vi "tabRecurser.vi"(4 "examineArrays?(T)":bool, 6 "Mode":enum16{"Read", "Write"}(ring)=enum."Write", 7 "controlsOnly":bool, 9 "SectionNameIn":string, 10 "controlsIn[]":refnum<vi>[](array[refnum]), 11 "INIrefnumIn":T3) -> (1 "varDescriptions":T1[](array[typedef]), 3 "INIrefnumOut":T3)   [LabVIEW 2021]
uses:
  <vilib>/Utility/config.llb/Config Data RefNum.ctl
  varDescriptor.ctl
  <vilib>/Utility/Data Type/Type Definitions/Data Type.ctl
  <vilib>/Utility/Data Type/NI_Data Type.lvlib
  <vilib>/Utility/config.llb/NI_LVConfig.lvlib
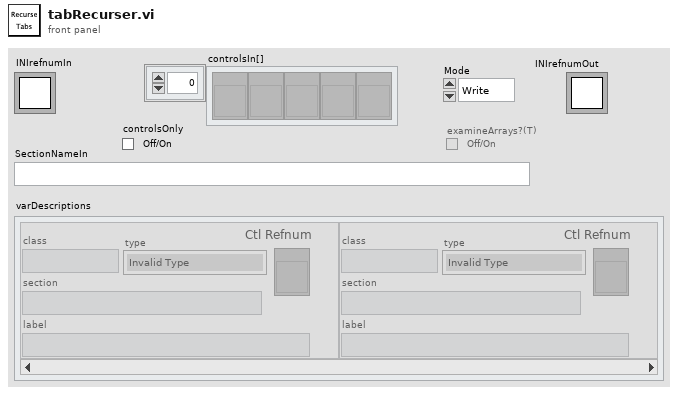
[diagram p1: front panel]
types:
  T1 = typedef "varDescriptor.ctl" = cluster{"class":string, "type":T2, "section":string, "label":string, "Ctl Refnum":refnum<vi>}
  T2 = typedef "NI_Data Type.lvlib/Data Type.ctl" = enum8{"Invalid Type", "Void", "I8", "I16", "I32", "I64", "U8", "U16", "U32", "U64", "Single Float", "Double Float", "Extended Float", "Single Complex", "Double Complex", "Extended Complex", "Enum U8", "Enum U16", "Enum U32", "Enum U64", "Single Float With Unit", "Double Float With Unit", "Extended Float With Unit", "Single Complex with Unit", "Double Complex with Unit", "Extended Complex with Unit", "Boolean", "String", "Path", "Picture", "Tag", "Array", "Cluster", "Variant", "LV Variant", "Waveform", "Timestamp", "Digital Waveform", "Digital Data", "ExpressData", "Refnum", "External Data", "VI", "Poly VI", "LabVIEW Class Instance", "Fixed Point", "Set Collection", "Map Collection"}
  T3 = typedef "NI_LVConfig.lvlib/Config Data RefNum.ctl" = refnum<k1>
  T4 = cluster{"ClassName":string, "type":T2, "SectionNameIn":string, "name":string, refnum<vi>}
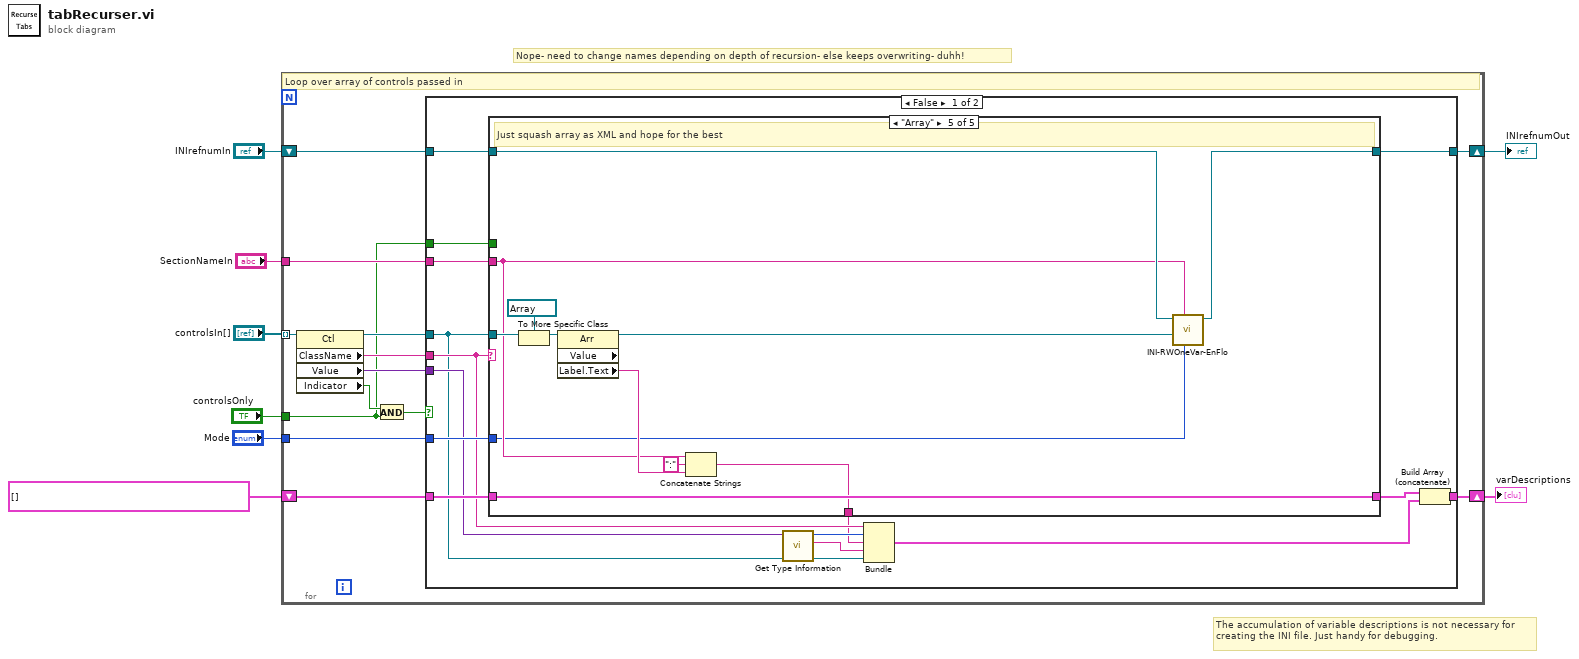
[diagram p0: block diagram]
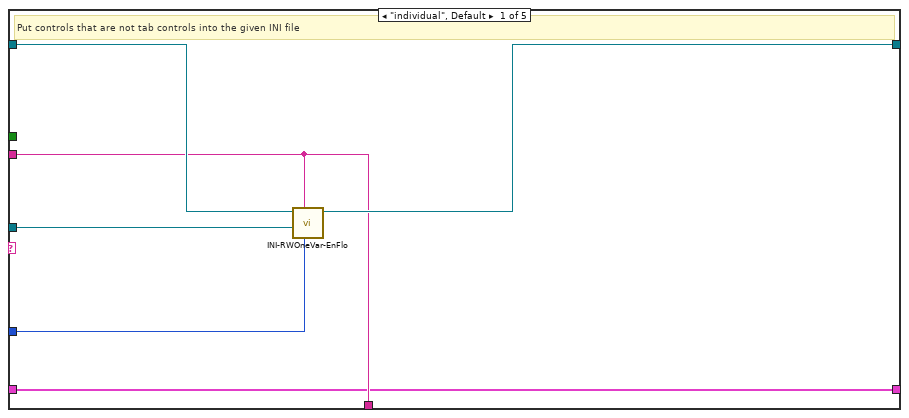
[diagram p2: hidden frame]
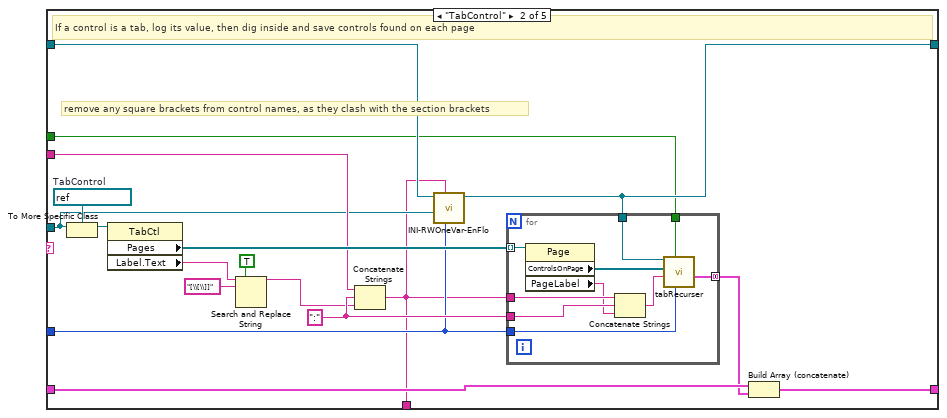
[diagram p3: hidden frame]
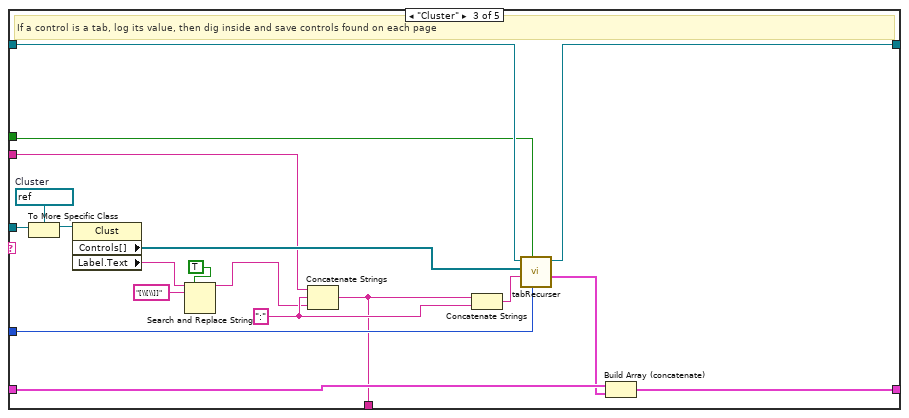
[diagram p4: hidden frame]
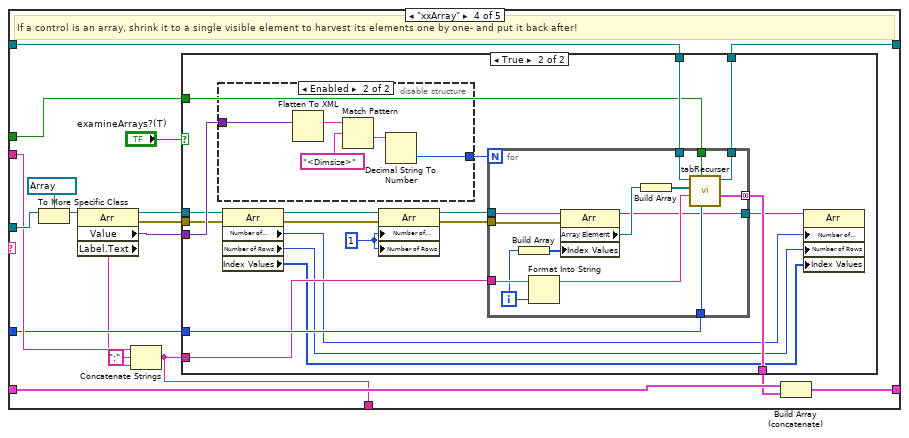
[diagram p5: hidden frame]
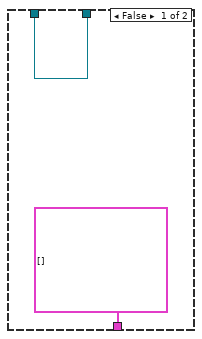
[diagram p6: hidden frame]
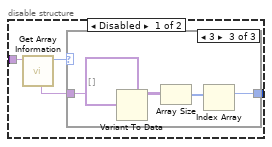
[diagram p7: hidden frame]
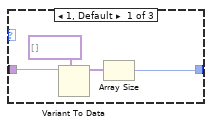
[diagram p8: hidden frame]
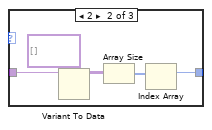
[diagram p9: hidden frame]
diagram:
  # "Nope- need to change names depending on depth of recursion- else keeps overwriting- duhh!"
  # "The accumulation of variable descriptions is not necessary for creating the INI file. Just handy for debugging."
  n1 = for {
    tunnel: "controlsIn[]" -> [w21] mode=indexing
    shift-right: [w13] -> w3
    shift-left: T1[] [] ("Array 2") -> [w20]
    tunnel: "SectionNameIn" -> [w19]
    shift-right: [w17] -> w5
    shift-left: "INIrefnumIn" -> [w18]
    tunnel: "Mode" -> [w16]
    tunnel: "controlsOnly" -> [w9]
    # "Loop over array of controls passed in"
    n2 = property class="Ctl"(reference=w21) -> (reference out=w12:refnum<vi>, "ClassName"=w14:string, "Value"=w15:variant, "Indicator"=w11:bool)  [unwired: 1 in, 1 out]
    n3 = And(x=w11, y=w9) -> (x .and. y?=w10:bool)
    n4 = case shown="False" w10 {
      tunnel: w20 -> [w35 w177]
      tunnel: w19 -> [w34 _]
      tunnel: w18 -> [w33 w178]
      tunnel: [w32 w178] -> w17
      tunnel: w16 -> [w31 _]
      tunnel: w15 -> [w28 _]
      tunnel: w14 -> [w27 _]
      tunnel: [w26 w177] -> w13
      tunnel: w12 -> [w24 _]
      tunnel: w9 -> [w22 _]
      frame False {
        n5 = case shown="\"Array\"" w27 {
          tunnel: w24 -> [w42 w52 w80 w106 w175]
          tunnel: [w37 w59 w88 w104 w174] -> w36
          tunnel: w35 -> [w37 w60 w89 w105 w174]
          tunnel: w34 -> [w38 w55 w83 w102 w167]
          tunnel: w33 -> [w41 w53 w81 w100 w172]
          tunnel: [w40 w48 w84 w98 w171] -> w32
          tunnel: w31 -> [w39 w51 w79 w101 w165]
          tunnel: [w38 w49 w77 w97 w170] -> w23
          tunnel: w22 -> [_ w43 w71 w90 _]
          frame "individual", Default {
            # "Put controls that are not tab controls into the given INI file"
            n6 = call "INI-RWOneVar-EnFlo.vi"("Mode"=w39, "section"=w38, "controlRefIn"=w42, "INIfileRefIn"=w41) -> ("INIfileRefOut"=w40:T3)  [unwired: 6 in, 1 out]
          }
          frame "TabControl" {
            w54 = ":" ("string")
            w56 = refnum<vi> refnum  # TabControl
            # "remove any square brackets from control names, as they clash with the section brackets"
            # "If a control is a tab, log its value, then dig inside and save controls found on each page"
            n7 = To More Specific Class(target class=w56, reference=w52) -> (specific class reference=w58:refnum<vi>)  [unwired: 1 in, 1 out]
            n8 = property class="TabCtl"(reference=w58) -> ("Pages"=w57:refnum<vi>[], "Label.Text"=w46:string)  [unwired: 1 in, 2 out]
            n9 = Search and Replace String(replace all?=TRUE ("replace all? (F)"), input string=w46, search string="[\\[\\]]") -> (result string=w45:string)  [unwired: 5 in, 3 out]
            n10 = Concatenate Strings(w55, w54, w45) -> (w49:string)
            n11 = call "INI-RWOneVar-EnFlo.vi"("Mode"=w51, "section"=w49, "controlRefIn"=w52, "INIfileRefIn"=w53) -> ("INIfileRefOut"=w48:T3)  [unwired: 6 in, 1 out]
            n12 = for {
              tunnel: w57 -> [w70] mode=indexing
              tunnel: w49 -> [w66]
              tunnel: w48 -> [w68]
              tunnel: w51 -> [w67]
              tunnel: w54 -> [w65]
              tunnel: [w62] -> w50 mode=concatenating
              tunnel: w43 -> [w61]
              n13 = property class="Page"(reference=w70) -> ("ControlsOnPage"=w69:refnum<vi>[], "PageLabel"=w64:string)  [unwired: 1 in, 2 out]
              n14 = Concatenate Strings(w66, w65, w64) -> (w63:string)
              n15 = call "tabRecurser.vi"("Mode"=w67, "controlsOnly"=w61, "SectionNameIn"=w63, "controlsIn[]"=w69, "INIrefnumIn"=w68) -> ("varDescriptions"=w62:T1[])  [unwired: 5 in, 1 out]
            }
            n16 = Build Array (concatenate)(w60, w50) -> (w59:T1[])
          }
          frame "Cluster" {
            w82 = ":" ("string")
            w85 = refnum<vi> refnum  # Cluster
            # "If a control is a tab, log its value, then dig inside and save controls found on each page"
            n17 = To More Specific Class(target class=w85, reference=w80) -> (specific class reference=w87:refnum<vi>)  [unwired: 1 in, 1 out]
            n18 = property class="Clust"(reference=w87) -> ("Controls[]"=w86:refnum<vi>[], "Label.Text"=w73:string)  [unwired: 1 in, 2 out]
            n19 = Search and Replace String(replace all?=TRUE ("replace all? (F)"), input string=w73, search string="[\\[\\]]") -> (result string=w72:string)  [unwired: 5 in, 3 out]
            n20 = Concatenate Strings(w83, w82, w72) -> (w77:string)
            n21 = Concatenate Strings(w77, w82) -> (w76:string)
            n22 = call "tabRecurser.vi"("Mode"=w79, "controlsOnly"=w71, "SectionNameIn"=w76, "controlsIn[]"=w86, "INIrefnumIn"=w81) -> ("varDescriptions"=w78:T1[], "INIrefnumOut"=w84:T3)  [unwired: 5 in]
            n23 = Build Array (concatenate)(w89, w78) -> (w88:T1[])
          }
          frame "xxArray" {
            # "If a control is an array, shrink it to a single visible element to harvest its elements one by one- and put it back after!"
            n24 = To More Specific Class(target class=refnum<vi> refnum ("Cluster-Array"), reference=w106) -> (specific class reference=w96:refnum<vi>)  [unwired: 1 in, 1 out]
            n25 = property class="Arr"(reference=w96) -> (reference out=w93:refnum<vi>, error out=w92:errorcluster, "Value"=w94:variant, "Label.Text"=w95:string)  [unwired: 1 in]
            n26 = Concatenate Strings(w102, ":" ("string"), w95) -> (w97:string)
            n27 = case shown="True" "examineArrays?(T)" {
              tunnel: w101 -> [_ w128]
              tunnel: w100 -> [w109 w127]
              tunnel: [T1[] [] ("varDescriptions") w126] -> w99
              tunnel: [w109 w125] -> w98
              tunnel: w97 -> [_ w124]
              tunnel: w94 -> [_ w122]
              tunnel: w93 -> [_ w121]
              tunnel: w92 -> [_ w118]
              tunnel: w90 -> [_ w110]
              frame False {
              }
              frame True {
                w115 = u32 1 ("Number of Columns")
                n28 = disable-structure shown="Enabled" {
                  disable-tunnel: [w131 w146] -> w123
                  disable-tunnel: w122 -> [w130 w147]
                  frame Disabled {
                    n29 = call <vilib>:"Get Array Information.vi"("variant"=w130) -> ("number of dimensions"=w129:i32)  [unwired: 7 in, 3 out]
                    n30 = case shown="3" w129 {
                      tunnel: w130 -> [w134 w139 w144]
                      tunnel: [w132 w136 w141] -> w131
                      frame 1, Default {
                        n31 = Variant To Data(type=variant[] [], Variant=w134) -> (data=w133:variant[])  [unwired: 1 in, 1 out]
                        n32 = Array Size(array=w133) -> (size(s)=w132:i32)
                      }
                      frame 2 {
                        n33 = Variant To Data(type=variant[][] [], Variant=w139) -> (data=w138:variant[][])  [unwired: 1 in, 1 out]
                        n34 = Array Size(array=w138) -> (size(s)=w137:i32[])
                        n35 = Index Array(array=w137) -> (element=w136:i32)  [unwired: 1 in]
                      }
                      frame 3 {
                        n36 = Variant To Data(type=variant[][][] [], Variant=w144) -> (data=w143:variant[][][])  [unwired: 1 in, 1 out]
                        n37 = Array Size(array=w143) -> (size(s)=w142:i32[])
                        n38 = Index Array(array=w142) -> (element=w141:i32)  [unwired: 1 in]
                      }
                    }
                  }
                  frame Enabled {
                    n39 = Flatten To XML(6:w147) -> (2:w148:string)
                    n40 = Match Pattern(string=w148, regular expression="<Dimsize>") -> (after substring=w150:string)  [unwired: 1 in, 3 out]
                    n41 = Decimal String To Number(string=w150) -> (number=w146:i32)  [unwired: 2 in, 1 out]
                  }
                }
                n42 = property class="Arr"(reference=w121, error in=w118) -> (reference out=w120:refnum<vi>, error out=w119:errorcluster, "Number of Columns"=w113:u32, "Number of Rows"=w112:u32, "Index Values"=w111:u32[])
                n43 = property class="Arr"(reference=w120, error in=w119, "Number of Columns"=w115, "Number of Rows"=w115) -> (reference out=w117:refnum<vi>, error out=w116:errorcluster)
                n44 = for {
                  N: w123 -> [_]
                  tunnel: w116 -> [w156]
                  tunnel: w117 -> [w157]
                  tunnel: w128 -> [w164]
                  tunnel: w127 -> [w163]
                  tunnel: [w162] -> w126 mode=concatenating
                  tunnel: [w161] -> w125
                  tunnel: w124 -> [w160]
                  tunnel: [w152] -> w114
                  tunnel: w110 -> [w151]
                  i -> [w155]
                  n45 = Build Array(w155) -> (w154:i32[])
                  n46 = Format Into String(initial string=w160, w155) -> (resulting string=w159:string)  [unwired: 2 in, 1 out]
                  n47 = property class="Arr"(reference=w157, error in=w156, "Index Values"=w154) -> (reference out=w152:refnum<vi>, "Array Element"=w153:refnum<vi>)  [unwired: 1 out]
                  n48 = Build Array(w153) -> (w158:refnum<vi>[])
                  n49 = call "tabRecurser.vi"("Mode"=w164, "controlsOnly"=w151, "SectionNameIn"=w159, "controlsIn[]"=w158, "INIrefnumIn"=w163) -> ("varDescriptions"=w162:T1[], "INIrefnumOut"=w161:T3)  [unwired: 5 in]
                }
                n50 = property class="Arr"(reference=w114, "Number of Columns"=w113, "Number of Rows"=w112, "Index Values"=w111) -> ()  [unwired: 1 in, 2 out]
              }
            }
            n51 = Build Array (concatenate)(w105, w99) -> (w104:T1[])
          }
          frame "Array" {
            # "Just squash array as XML and hope for the best"
            n52 = To More Specific Class(target class=refnum<vi> refnum ("Cluster-Array"), reference=w175) -> (specific class reference=w169:refnum<vi>)  [unwired: 1 in, 1 out]
            n53 = property class="Arr" props=["Value", "Label", "Text"](reference=w169) -> (reference out=w166:refnum<vi>, "Label.Text"=w168:string)  [unwired: 1 in, 2 out]
            n54 = Concatenate Strings(w167, ":" ("string"), w168) -> (w170:string)
            n55 = call "INI-RWOneVar-EnFlo.vi"("Mode"=w165, "section"=w167, "controlRefIn"=w166, "INIfileRefIn"=w172) -> ("INIfileRefOut"=w171:T3)  [unwired: 6 in, 1 out]
          }
        }
        n56 = call <vilib>:"Get Type Information.vi"("variant"=w28) -> ("name"=w29:string, "type"=w30:T2)  [unwired: 6 in, 3 out]
        n57 = Bundle("ClassName"=w27, "type"=w30, "SectionNameIn"=w23, "name"=w29, w24) -> (w25:T4)  [unwired: 1 in]
        n58 = Build Array (concatenate)(w36, w25) -> (w26:T1[])
      }
      frame True {
      }
    }
  }
  "INIrefnumOut" <- w5
  "varDescriptions" <- w3
